vi "2020_day09.vi"() -> ()   [LabVIEW 2021]
panel:
  out "Task 2 (outlier)":i32
  out "Task 1 (outlier)":i32
  in  "Switch":bool caption="Ex. Data  vs.  User Data"
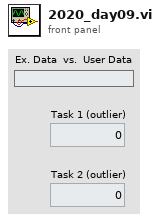
[diagram p1: front panel]
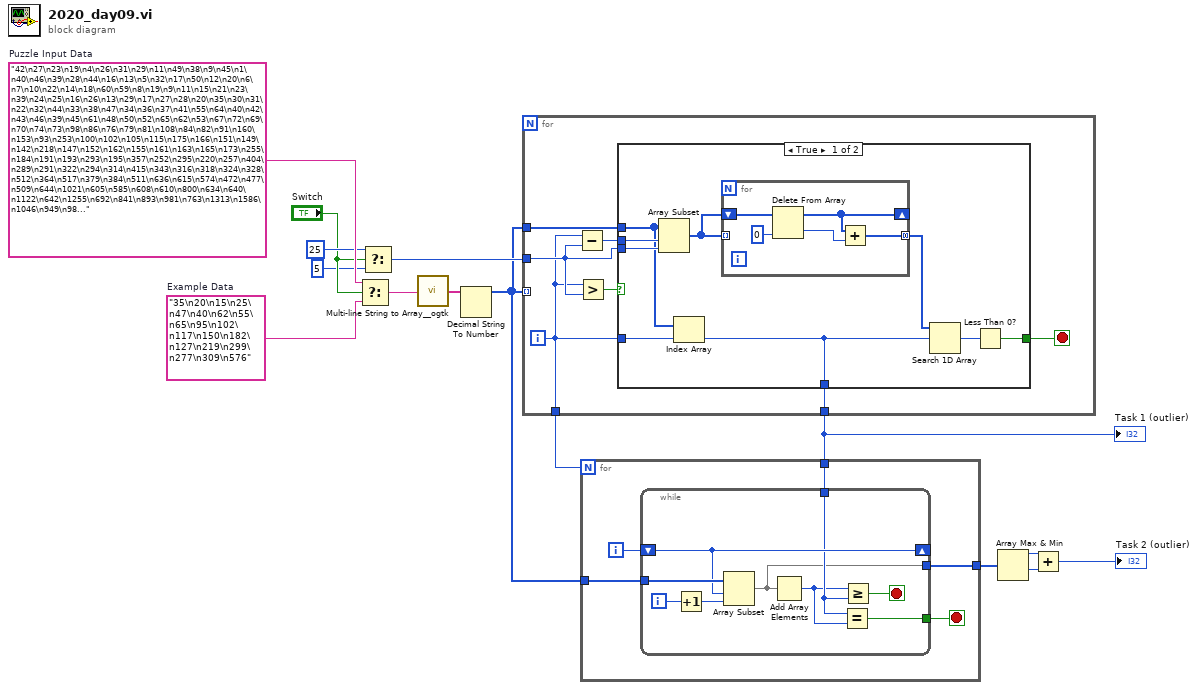
[diagram p0: block diagram]
diagram:
  w14 = "42\n27\n23\n19\n4\n26\n31\n29\n11\n49\n38\n9\n45\n1\n40\n46\n39\n28\n44\n16\n13\n5\n32\n17\n50\n12\n20\n6\n7\n10\n22\n14\n18\n60\n59\n8\n19\n9\n11\n15\n21\n23\n39\n24\n25\n16\n26\n13\n29\n17\n27\n28\n20\n35\n30\n31\n22\n32\n44\n33\n38\n47\n34\n36\n37\n41\n55\n64\n40\n42\n43\n46\n39\n45\n61\n48\n50\n52\n65\n62\n53\n67\n72\n69\n70\n74\n73\n98\n86\n76\n79\n81\n108\n84\n82\n91\n160\n153\n93\n253\n100\n102\n105\n115\n175\n166\n151\n149\n142\n218\n147\n152\n162\n155\n161\n163\n165\n173\n255\n184\n191\n193\n293\n195\n357\n252\n295\n220\n257\n404\n289\n291\n322\n294\n314\n415\n343\n316\n318\n324\n328\n512\n364\n517\n379\n384\n511\n636\n615\n574\n472\n477\n509\n644\n1021\n605\n585\n608\n610\n800\n634\n640\n1122\n642\n1255\n692\n841\n893\n981\n763\n1313\n1586\n1046\n949\n98..."  # Puzzle Input Data
  w15 = "35\n20\n15\n25\n47\n40\n62\n55\n65\n95\n102\n117\n150\n182\n127\n219\n299\n277\n309\n576"  # Example Data
  n1 = Select(t=w14, s="Switch", f=w15) -> (s? t:f=w13:string)
  n2 = Select(t=25 ("y"), s="Switch", f=5 ("y")) -> (s? t:f=w8:i32)
  n3 = call <userlib>:"Multi-line String to Array__ogtk.vi"("string"=w13) -> ("lines"=w12:string[])
  n4 = Decimal String To Number(string=w12) -> (number=w7:i32[])  [unwired: 2 in, 1 out]
  n5 = for {
    tunnel: w7 -> [_] mode=indexing
    tunnel: w7 -> [w22]
    tunnel: w8 -> [w19]
    tunnel: [w17] -> w6
    tunnel: [w16] -> w5
    i -> [w17]
    stop <- w20 stop-if-true
    n6 = Subtract(x=w17, y=w19) -> (x-y=w21:i32)
    n7 = Greater?(x=w17, y=w19) -> (0:w18:bool)
    n8 = case shown="True" w18 {
      tunnel: w22 -> [w28 _]
      tunnel: w21 -> [w31 _]
      tunnel: w19 -> [w30 _]
      tunnel: [w25 _] -> w20
      tunnel: w17 -> [w24 _]
      tunnel: [w23 _] -> w16
      frame True {
        n9 = Array Subset(array=w28, index=w31, length=w30) -> (w29:i32[])
        n10 = Index Array(array=w28, index=w24) -> (element=w23:i32)
        n11 = for {
          tunnel: w29 -> [_] mode=indexing
          shift-right: [w35] -> _
          shift-left: w29 -> [w36]
          tunnel: [w33] -> w27 mode=concatenating
          n12 = Delete From Array(array=w36, index=0) -> (deleted portion=w34:i32, array with subset deleted=w35:i32[])  [unwired: 1 in]
          n13 = Add(x=w35, y=w34) -> (x+y=w33:i32[])
        }
        n14 = Search 1D Array(1D array=w27, element=w23) -> (index of element=w26:i32)  [unwired: 1 in]
        n15 = Less Than 0?(x=w26) -> (x < 0?=w25:bool)
      }
      frame False {
      }
    }
  }
  "Task 1 (outlier)" <- w5
  n16 = for {
    N: w6 -> [_]
    tunnel: w7 -> [w41]
    tunnel: w5 -> [w39]
    tunnel: [w37] -> w4
    i -> [w40]
    stop <- w38 stop-if-true
    n17 = while {
      tunnel: w41 -> [w50]
      shift-right: [w49] -> _
      shift-left: w40 -> [w49]
      tunnel: w39 -> [w45]
      tunnel: [w43] -> w38
      tunnel: [w42] -> w37
      i -> [w48]
      stop <- w46 stop-if-true
      n18 = Increment(x=w48) -> (x+1=w47:i32)
      n19 = Array Subset(array=w50, index=w49, length=w47) -> (w42:i32[])
      n20 = Add Array Elements(numeric array=w42) -> (sum=w44:i32)
      n21 = Equal?(x=w45, y=w44) -> (x = y?=w43:bool)
      n22 = Greater Or Equal?(x=w44, y=w45) -> (x >= y?=w46:bool)
    }
  }
  n23 = Array Max & Min(array=w4) -> (max value=w3:i32, min value=w2:i32)  [unwired: 2 out]
  n24 = Add(x=w3, y=w2) -> (x+y=→"Task 2 (outlier)":i32)
